vi "Get Name.vi"(8 "error in (no error)":errorcluster, 11 "Workstation in":refnum<class "Workstation.lvclass">) -> (0 "error out":errorcluster, 2 "Name":string, 3 "Workstation out":refnum<class "Workstation.lvclass">)   [LabVIEW 2020, in "Workstation.lvclass"]
uses:
  Workstation.lvclass
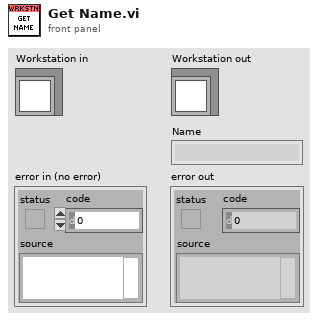
[diagram p1: front panel]
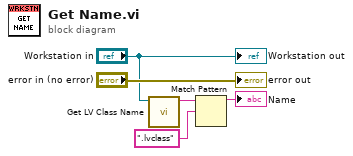
[diagram p0: block diagram]
diagram:
  n1 = call <vilib>:"Get LV Class Name.vi"("object"="Workstation in") -> ("class name"=w4:string)  [unwired: 9 in, 1 out]
  n2 = Match Pattern(string=w4, regular expression=".lvclass") -> (before substring=→"Name":string)  [unwired: 1 in, 3 out]
  "error out" <- "error in (no error)"
  "Workstation out" <- "Workstation in"
